vi "Get Available Software 1.0.vi"   [LabVIEW 2014, in "nisyscfg.lvlib"]
doc: "Retrieves a list of software available on the local system."
uses:
  nisyscfg.lvlib
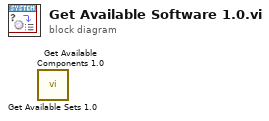
[diagram p0: block diagram]
diagram:
  n1 = call "Get Available Sets 1.0.vi"() -> ()  [unwired: 9 in, 3 out]
  n2 = call "Get Available Components 1.0.vi"() -> ()  [unwired: 9 in, 3 out]
